vi "Choose Tag.vi"(7 "DC Overvoltage":bool, 10 "Frame Tag Bypass":T2, 11 "Line Status In":T4) -> (0 "Frame Count":u32, 2 "Frametag Data":T1, 3 "Send Tag":bool)   [LabVIEW 2014]
uses:
  Acquisition Engine/Acquisition Status.ctl
  Async Frametag Data.ctl
  Frametag Data.ctl
panel:
  # "Copyright 2014 Vidrio Technologies\nScanImage 5 software is licensed under the Apache License, Version 2.0 (the \"License\"); you may not use any files contained\nwithin the ScanImage 5 release except in compliance with the License. You may obtain a copy of the License at\n http://www.apache.org/licenses/LICENSE-2.0\nUnless required by applicable law or agreed to in writing, software distributed under the License is distributed on an\n\"AS IS\" BASIS, WITHOUT WARRANTIES OR CONDITIONS OF ANY KIND, either express or implied. See the License for the\n specific language governing permissions and limitations under the License."
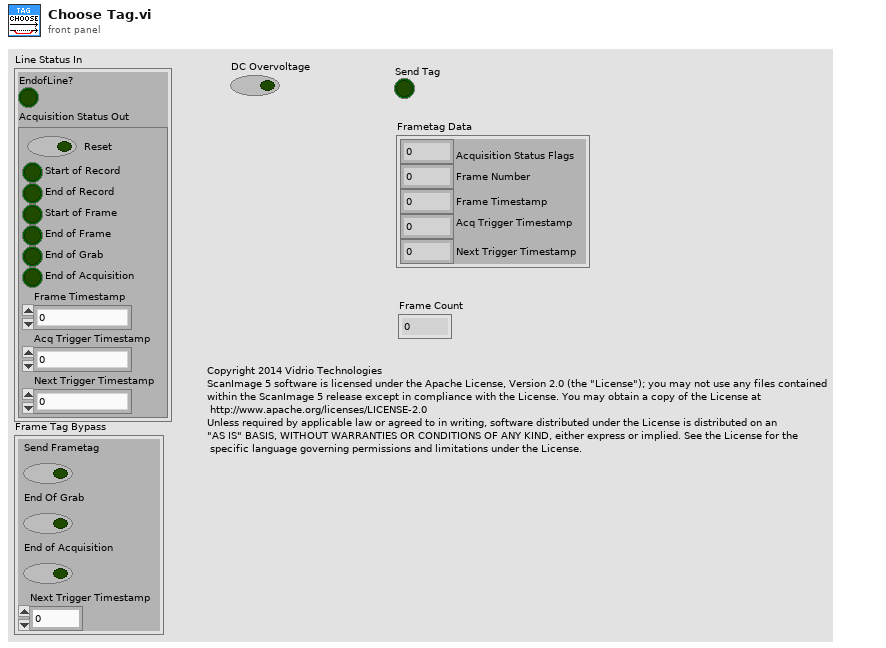
[diagram p1: front panel]
types:
  T1 = typedef "Frametag Data.ctl" = cluster{"Acquisition Status Flags":u16, "Frame Number":u32, "Frame Timestamp":u64, "Acq Trigger Timestamp":u64, "Next Trigger Timestamp":u64}
  T2 = typedef "Async Frametag Data.ctl" = cluster{"Send Frametag":bool, "End Of Grab":bool, "End of Acquisition":bool, "Next Trigger Timestamp":u64}
  T3 = typedef "Acquisition Status.ctl" = cluster{"Reset":bool, "Start of Record":bool, "End of Record":bool, "Start of Frame":bool, "End of Frame":bool, "End of Grab":bool, "End of Acquisition":bool, "Frame Timestamp":u64, "Acq Trigger Timestamp":u64, "Next Trigger Timestamp":u64}
  T4 = cluster{"EndofLine?":bool, "Acquisition Status Out":T3}
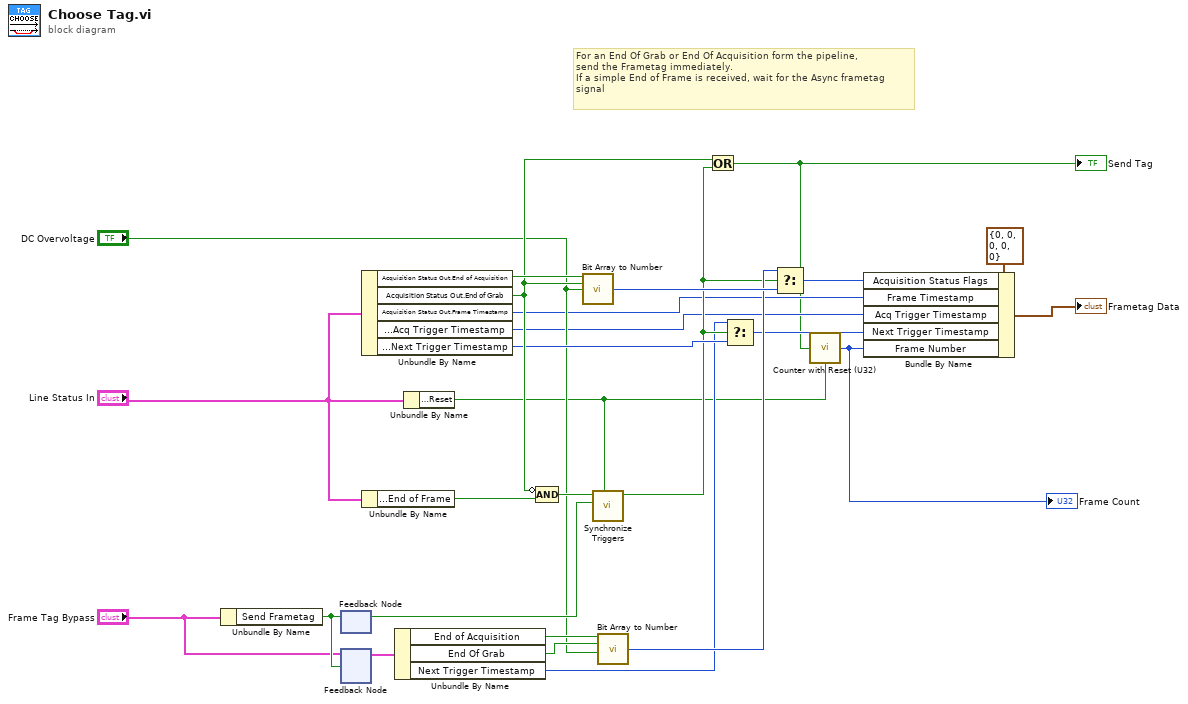
[diagram p0: block diagram]
diagram:
  # "For an End Of Grab or End Of Acquisition form the pipeline,\nsend the Frametag immediately.\nIf a simple End of Frame is received, wait for the Async frametag\nsignal"
  n1 = Unbundle By Name("Frame Tag Bypass") -> ("Send Frametag"=w14:bool)
  n2 = feedback #1() -> (w13:bool)  [unwired: 1 in]
  n3 = feedback-in #1(w14) -> ()
  n4 = feedback #2() -> (w24:T2)  [unwired: 1 in]
  n5 = feedback-in #2("Frame Tag Bypass", w14) -> ()
  n6 = Unbundle By Name("Line Status In") -> ("Acquisition Status Out.End of Acquisition"=w26:bool, "Acquisition Status Out.End of Grab"=w22:bool, "Acquisition Status Out.Frame Timestamp"=w7:u64, "Acquisition Status Out.Acq Trigger Timestamp"=w6:u64, "Acquisition Status Out.Next Trigger Timestamp"=w17:u64)
  n7 = Unbundle By Name("Line Status In") -> ("Acquisition Status Out.End of Frame"=w23:bool)
  n8 = Unbundle By Name(w24) -> ("End of Acquisition"=w21:bool, "End Of Grab"=w20:bool, "Next Trigger Timestamp"=w15:u64)
  n9 = Unbundle By Name("Line Status In") -> ("Acquisition Status Out.Reset"=w2:bool)
  n10 = Compound Arithmetic op=AND(invert w22, w23) -> (w25:bool)
  n11 = call "Bit Array to Number.vi"("Bit 0"=w26, "Bit 1"=w22, "Bit 2"="DC Overvoltage") -> ("flags"=w19:u16)  [unwired: 12 in]
  n12 = call "Synchronize Triggers.vi"("Reset"=w2, "In2"=w13, "In1"=w25) -> ("Out"=w16:bool)  [unwired: 8 in]
  n13 = call "Bit Array to Number.vi"("Bit 0"=w21, "Bit 1"=w20, "Bit 2"="DC Overvoltage") -> ("flags"=w18:u16)  [unwired: 12 in]
  n14 = Or(x=w22, y=w16) -> (x .or. y?=w3:bool)
  "Send Tag" <- w3
  n15 = Select(t=w15, s=w16, f=w17) -> (s? t:f=w5:u64)
  n16 = Select(t=w18, s=w16, f=w19) -> (s? t:f=w8:u16)
  n17 = call "Counter with Reset (U32).vi"("Reset?"=w2, "Increment"=w3) -> ("Counter"=w1:u32)  [unwired: 13 in]
  "Frame Count" <- w1
  n18 = Bundle By Name(cluster=T1 {"Acquisition Status Flags"=0, "Frame Number"=0, "Frame Timestamp"=0, "Acq Trigger Timestamp"=0, "Next Trigger Timestamp"=0} ("TagData"), "Acquisition Status Flags"=w8, "Frame Timestamp"=w7, "Acq Trigger Timestamp"=w6, "Next Trigger Timestamp"=w5, "Frame Number"=w1) -> (→"Frametag Data":T1)
